vi "Write Active Channel.vi"(8 "error in (no error)":errorcluster, 10 "Active Channel":u32, 11 "Analog-Output in":refnum<class "Analog-Output.lvclass">) -> (0 "error out":errorcluster, 3 "Analog-Output out":refnum<class "Analog-Output.lvclass">)   [LabVIEW 2019, in "Analog-Output.lvlib" / "Analog-Output.lvclass"]
uses:
  Library/Analog-Output.lvclass
  C:/Users/Public/Documents/Development/builds/Instruments/Instruments.lvlibp/Library/Instruments.lvclass
  Library/Analog-Output.lvclass/Analog-Output.ctl
  builds/Instruments/Instruments.lvlibp/Private/Polymorphic/Special/Event from String.vi
  builds/Instruments/Instruments.lvlibp/Accessors/Command with Logging.vi
  builds/Instruments/Instruments.lvlibp/Library/Instruments.lvclass
  builds/Instruments/Instruments.lvlibp
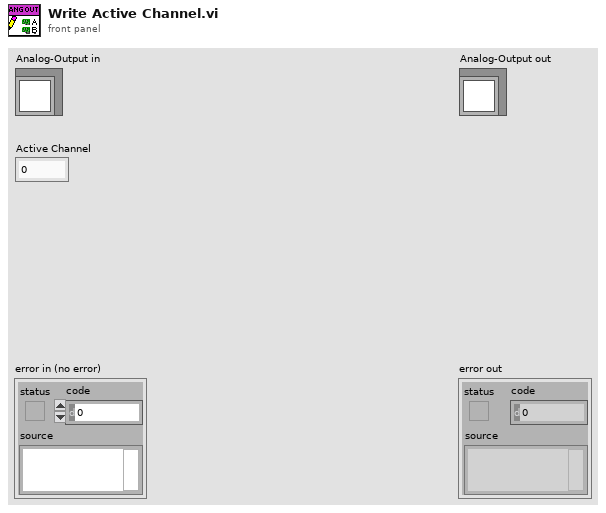
[diagram p1: front panel]
types:
  T1 = cluster{"Timestamp":timestamp, "Description":string, "Data":string}
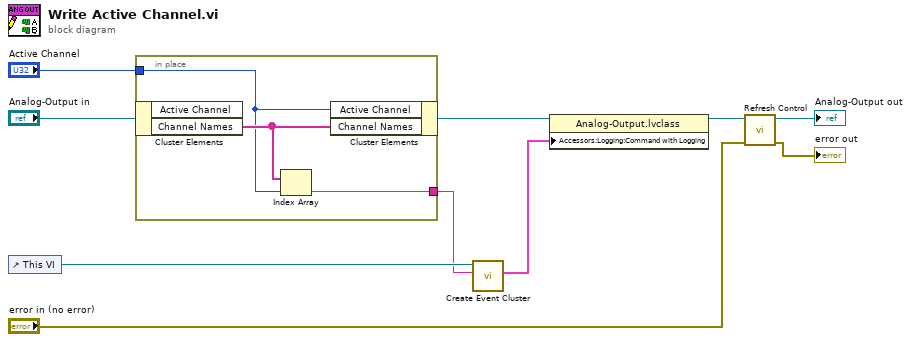
[diagram p0: block diagram]
diagram:
  n1 = control-ref of="This VI"() -> (w8:refnum<vi>)
  n2 = in-place {
    in-place-border: "Active Channel" -> [w12]
    in-place-border: [w11] -> w7
    n3 = in-place-cluster #1("Analog-Output in") -> ("Channel Names"=w13:string[])  [unwired: 1 out]
    n4 = Index Array(array=w13, index=w12) -> (element=w11:string)
    n5 = in-place-cluster #1("Active Channel"=w12, "Channel Names"=w13) -> (w6:refnum<class "Analog-Output.lvclass">)
  }
  n6 = call-poly "Create Event Cluster.vi"("Value"=w7, "VI Refnum"=w8) -> ("Event Data"=w5:T1)  [unwired: 9 in]
  n7 = property class="Analog-Output.lvclass"(reference=w6, "Accessors:Logging:Command with Logging"=w5) -> (reference out=w4:refnum<class "Analog-Output.lvclass">)  [unwired: 1 in, 1 out]
  n8 = call "Refresh Control.vi"("error in (no error)"="error in (no error)", "Analog-Output in"=w4) -> ("error out"=→"error out":errorcluster, "Analog-Output out"=→"Analog-Output out":refnum<class "Analog-Output.lvclass">)  [unwired: 8 in]
